vi "onListenForNewConnection.vi"(8 "error in (no error)":errorcluster, 9 "timeout (ms)":i32=1, 11 "Listener":refnum<class "Connection.lvclass">) -> (0 "error out":errorcluster, 1 "New connection":bool, 3 "New Connection":refnum<class "Connection.lvclass">)   [LabVIEW 2013, in "MQTT_Connection.lvlib" / "Connection.lvclass"]
uses:
  Connection.lvclass
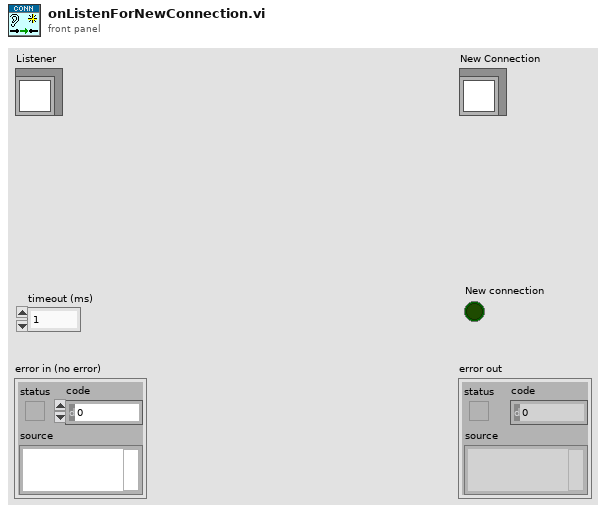
[diagram p1: front panel]
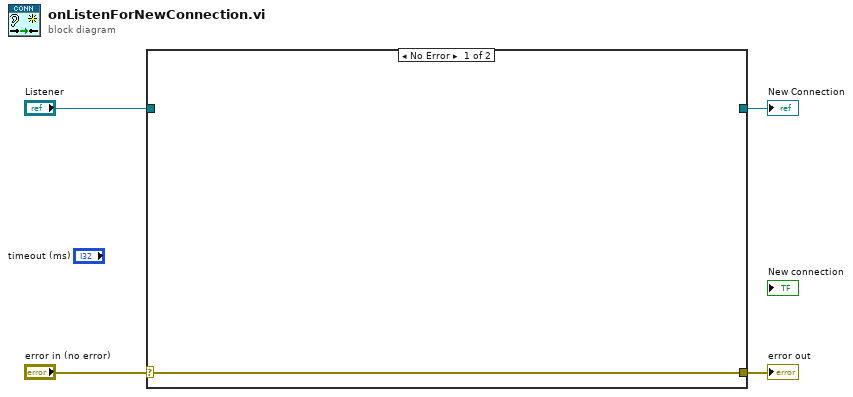
[diagram p0: block diagram]
diagram:
  n1 = case shown="No Error" "error in (no error)" {
    selector: "error in (no error)" -> [w5 w7]
    tunnel: [w5 w7] -> w3
    tunnel: [_ w6] -> w1
    tunnel: "Listener" -> [_ w6]
    frame No Error {
    }
    frame Error {
    }
  }
  "error out" <- w3
  "New Connection" <- w1
